vi "MasterCautionCalc.vi"(8 "All_Sensor_Readings":T1, 9 "All_Outputs":T5, 10 "All Driver Commands":T8) -> (3 "Master Caution":bool)   [LabVIEW 2012]
uses:
  TestProject/All_Commands.ctl
  TestProject/Cirular Shooter/circular_shooter_commands.ctl
  TestProject/Climber/Climber_Commands.ctl
  TestProject/All_Outputs.ctl
  TestProject/Cirular Shooter/Shooter_Outputs.ctl
  TestProject/Climber/Climber_Outputs.ctl
  TestProject/All_Sensor_Readings.ctl
  TestProject/Climber/climber_sensor_readings.ctl
  TestProject/Cirular Shooter/Shooter_inputs.ctl
  TestProject/Field Drive/Field_Drive_out.ctl
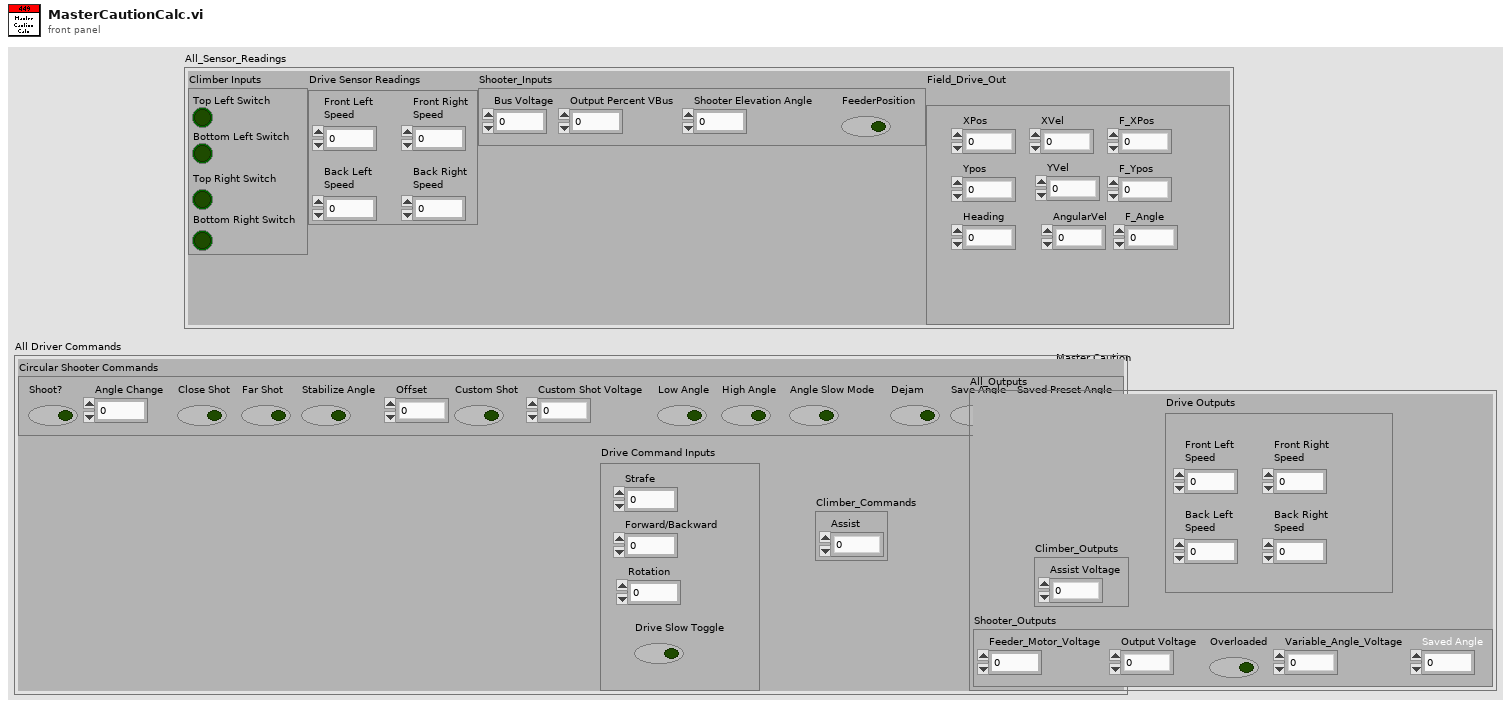
[diagram p1: front panel]
types:
  T1 = typedef "All_Sensor_Readings.ctl" = cluster{"Climber Inputs":T2, "Drive Sensor Readings":cluster{"Front Left\nSpeed":dbl, "Back Left\nSpeed":dbl, "Front Right\nSpeed":dbl, "Back Right\nSpeed":dbl}, "Shooter_Inputs":T3, "Field_Drive_Out\n":T4}
  T2 = typedef "climber_sensor_readings.ctl" = cluster{"Top Left Switch":bool, "Bottom Left Switch":bool, "Top Right Switch":bool, "Bottom Right Switch":bool}
  T3 = typedef "Shooter_inputs.ctl" = cluster{"Bus Voltage":dbl, "Output Percent VBus":dbl, "Shooter Elevation Angle":dbl, "FeederPosition":bool}
  T4 = typedef "Field_Drive_out.ctl" = cluster{"XPos":dbl, "Ypos":dbl, "XVel":dbl, "YVel":dbl, "Heading":dbl, "AngularVel":dbl, "F_XPos":dbl, "F_Ypos":dbl, "F_Angle":dbl}
  T5 = typedef "All_Outputs.ctl" = cluster{"Drive Outputs":cluster{"Front Left\nSpeed":dbl, "Back Left\nSpeed":dbl, "Front Right\nSpeed":dbl, "Back Right\nSpeed":dbl}, "Shooter_Outputs":T6, "Climber_Outputs":T7}
  T6 = typedef "Shooter_Outputs.ctl" = cluster{"Feeder_Motor_Voltage":dbl, "Output Voltage":dbl, "Overloaded":bool, "Variable_Angle_Voltage":dbl, "Saved Angle":dbl}
  T7 = typedef "Climber_Outputs.ctl" = cluster{"Assist Voltage":dbl}
  T8 = typedef "All_Commands.ctl" = cluster{"Circular Shooter Commands":T9, "Drive Command Inputs":cluster{"Strafe":dbl, "Forward/Backward":dbl, "Rotation":dbl, "Drive Slow Toggle":bool}, "Climber_Commands":T10}
  T9 = typedef "circular_shooter_commands.ctl" = cluster{"Shoot?":bool, "Angle Change":dbl, "Close Shot":bool, "Far Shot":bool, "Stabilize Angle ":bool, "Offset":dbl, "Custom Shot":bool, "Custom Shot Voltage":dbl, "Low Angle":bool, "High Angle":bool, "Angle Slow Mode":bool, "Dejam":bool, "Save Angle":bool, "Saved Preset Angle":bool}
  T10 = typedef "Climber_Commands.ctl" = cluster{"Assist":dbl}
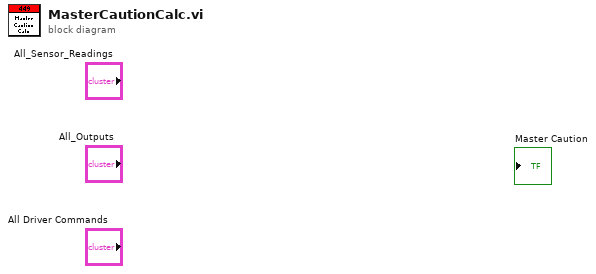
[diagram p0: block diagram]
diagram:
